vi "CRYProject Save & Load Scroll Manage.vi"(10 "StateLabel":string) -> ()   [LabVIEW 2013]
uses:
  CRYWindow/SubVI/CRYMain Sub Window Global.vi
  CRYProject Editor Global.vi
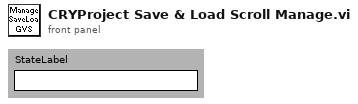
[diagram p1: front panel]
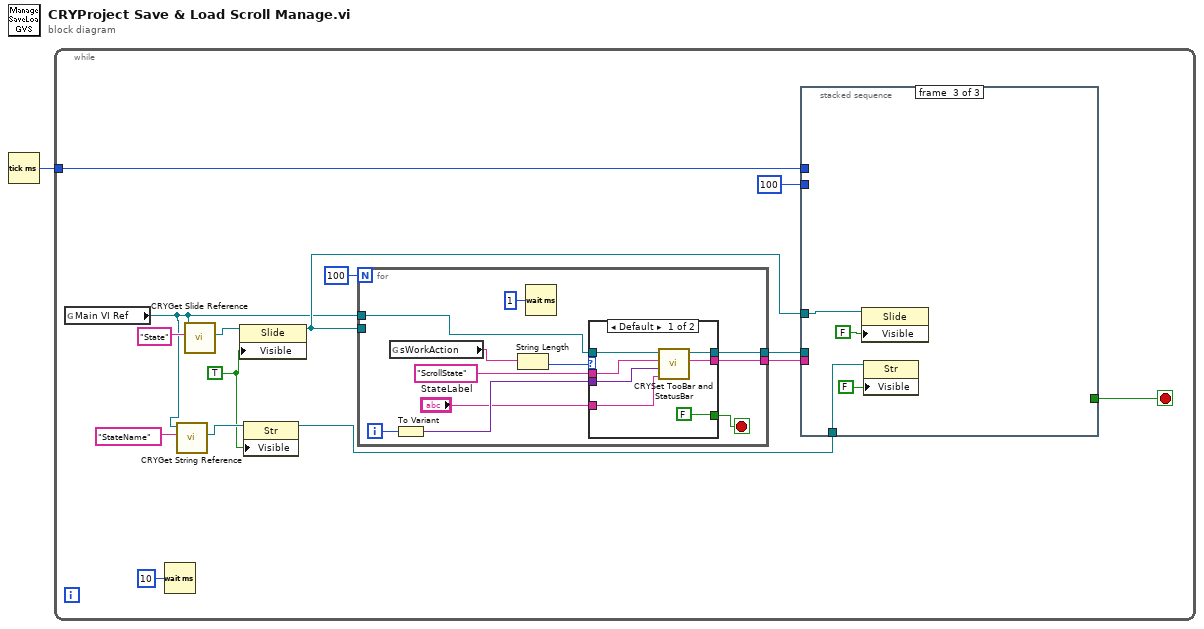
[diagram p0: block diagram]
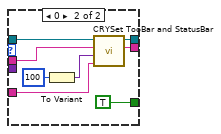
[diagram p2: hidden frame]
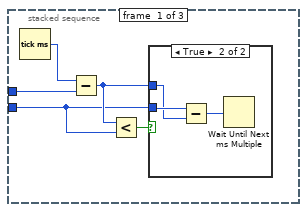
[diagram p3: hidden frame]
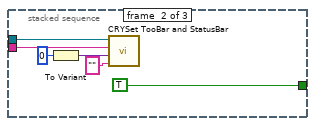
[diagram p5: hidden frame]
diagram:
  n1 = Tick Count (ms)() -> (millisecond timer value=w1:u32)
  n2 = while {
    tunnel: w1 -> [w8]
    stop <- w15 stop-if-true
    w3 = TRUE ("Visible")
    n3 = global read "CRYMain Sub Window Global.vi" "Main VI Ref"() -> (w4:refnum<vi>)
    n4 = Wait (ms)(milliseconds to wait=u32 10 ("millisecond multiple")) -> ()  [unwired: 1 out]
    n5 = call "CRYGet String Reference.vi"("Label Name"="StateName" ("Type"), "VI Refnum"=w4) -> ("String Ref Out"=w5:refnum<vi>)  [unwired: 7 in, 2 out]
    n6 = call "CRYGet Slide Reference.vi"("Label Name"="State" ("Type"), "VI Refnum"=w4) -> ("Slide Ref Out"=w10:refnum<vi>)  [unwired: 9 out]
    n7 = property class="Slide"(reference=w10, "Visible"=w3) -> (reference out=w9:refnum<vi>)  [unwired: 1 in, 1 out]
    n8 = property class="Str"(reference=w5, "Visible"=w3) -> (reference out=w2:refnum<vi>)  [unwired: 1 in, 1 out]
    n9 = for {
      N: 100 -> [_]
      tunnel: [w24] -> w13
      tunnel: [w23] -> w14
      tunnel: w9 -> [_]
      tunnel: w4 -> [w20]
      i -> [w27]
      stop <- w22 stop-if-true
      n10 = global read "CRYProject Editor Global.vi" "sWorkAction"() -> (w19:string)
      n11 = To Variant(anything=w27) -> (Variant=w25:variant)
      n12 = String Length(string=w19) -> (length=w18:i32)
      n13 = Wait (ms)(milliseconds to wait=u32 1) -> ()  [unwired: 1 out]
      n14 = case shown="Default" w18 {
        tunnel: w20 -> [w31 w36]
        tunnel: "ScrollState" ("Type") -> [w30 w35]
        tunnel: w25 -> [w32 _]
        tunnel: [w31 w36] -> w24
        tunnel: [w30 w35] -> w23
        tunnel: [FALSE TRUE] -> w22
        tunnel: "StateLabel" -> [w28 w33]
        frame Default {
          n15 = call "CRYSet TooBar and StatusBar.vi"("StateLabel"=w28, "variant"=w32, "Type"=w30, "MainVI Ref In"=w31) -> ()  [unwired: 8 out]
        }
        frame 0 {
          n16 = To Variant(anything=u8 100) -> (Variant=w37:variant)
          n17 = call "CRYSet TooBar and StatusBar.vi"("StateLabel"=w33, "variant"=w37, "Type"=w35, "MainVI Ref In"=w36) -> ()  [unwired: 8 out]
        }
      }
    }
    n18 = stacked-sequence {
      tunnel: w13 -> [_ w50 _]
      tunnel: w14 -> [_ w49 _]
      tunnel: [_ TRUE _] -> w15
      tunnel: w9 -> [_ _ w56]
      tunnel: w8 -> [w42 _ _]
      tunnel: 100 -> [w39 _ _]
      tunnel: w2 -> [_ _ w54]
      frame #0 {
        n19 = Tick Count (ms)() -> (millisecond timer value=w43:u32)
        n20 = Subtract(x=w43, y=w42) -> (x-y=w40:u32)
        n21 = Less?(x=w40, y=w39) -> (x < y?=w41:bool)
        n22 = case shown="True" w41 {
          tunnel: w40 -> [_ w45]
          tunnel: w39 -> [_ w46]
          frame False {
          }
          frame True {
            n23 = Subtract(x=w46, y=w45) -> (x-y=w44:u32)
            n24 = Wait Until Next ms Multiple(millisecond multiple=w44) -> ()  [unwired: 1 out]
          }
        }
      }
      frame #1 {
        n25 = To Variant(anything=u8 0) -> (Variant=w52:variant)
        n26 = call "CRYSet TooBar and StatusBar.vi"("StateLabel"="", "variant"=w52, "Type"=w49, "MainVI Ref In"=w50) -> ()  [unwired: 8 out]
      }
      frame #2 {
        n27 = property class="Slide"(reference=w56, "Visible"=FALSE) -> ()  [unwired: 1 in, 2 out]
        n28 = property class="Str"(reference=w54, "Visible"=FALSE) -> ()  [unwired: 1 in, 2 out]
      }
    }
  }
